vi "Car Go Down.vi"(9 "m array":i16[][](array[numeric]), 10 "Numeric":i32, 11 "Input in":i32[][](array[numeric])) -> (2 "move or not":bool, 3 "Input out":i32[][](array[numeric]))   [LabVIEW 2021]
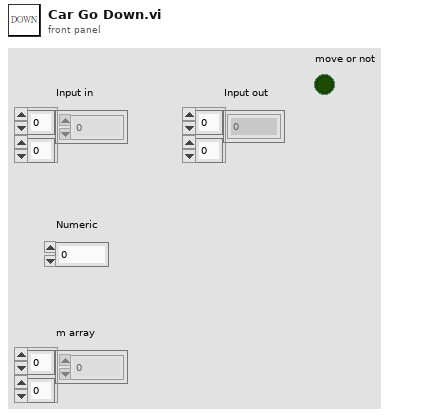
[diagram p1: front panel]
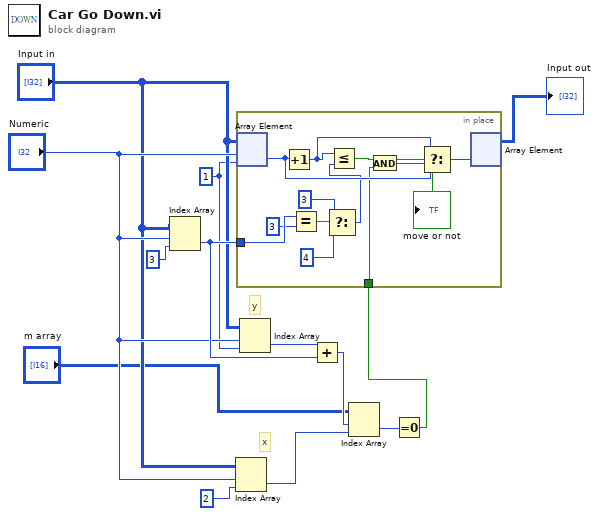
[diagram p0: block diagram]
diagram:
  w6 = 1
  # "x"
  # "y"
  n1 = Index Array(array="Input in", index (row)="Numeric", index (col)=3 ("disabled index (col)")) -> (element=w12:i32)
  n2 = Index Array(array="Input in", index (row)="Numeric", index (col)=2) -> (element=w4:i32)
  n3 = Index Array(array="Input in", index (row)="Numeric", index (col)=w6) -> (element=w11:i32)
  n4 = Add(x=w11, y=w12) -> (x+y=w13:i32)
  n5 = Index Array(array="m array", index (row)=w13, index (col)=w4) -> (element=w2:i16)
  n6 = Equal To 0?(x=w2) -> (x = 0?=w3:bool)
  n7 = in-place {
    in-place-border: w3 -> [w22]
    in-place-border: w12 -> [w21]
    n8 = in-place-array #1("Input in", "Numeric", w6) -> (w23:i32)
    n9 = Increment(x=w23) -> (x+1=w17:i32)
    n10 = Equal?(x=w21, y=3) -> (x = y?=w15:bool)
    n11 = Select(t=3, s=w15, f=4) -> (s? t:f=w16:i32)
    n12 = Less Or Equal?(x=w17, y=w16) -> (x <= y?=w25:bool)
    n13 = And(x=w25, y=w22) -> (x .and. y?=w14:bool)
    "move or not" <- w14
    n14 = Select(t=w17, s=w14, f=w23) -> (s? t:f=w24:i32)
    n15 = in-place-array #1(w24) -> (→"Input out":i32[][])  [unwired: 2 out]
  }
